vi "Quick Usb Bulk Data Stop Stream.vi"(8 "error in (no error)":errorcluster, 10 "wait":u8, 11 "hDevice":u32) -> (0 "error out":errorcluster, 2 "function return":i32, 3 "hDevice out":u32)   [LabVIEW 2011, in "QuickUSB.lvlib"]
doc: "QUSBLIB QRETURN QuickUsbBulkDataStopStream(\n QHANDLE hDevice,\n QBOOL wait\n);"
uses:
  QuickUSB.lvlib
  QuickUSB.dll
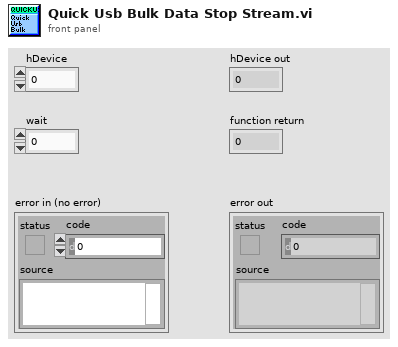
[diagram p1: front panel]
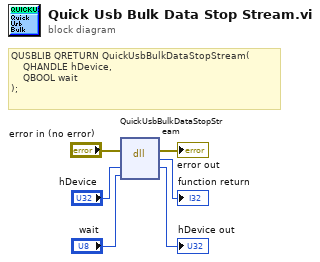
[diagram p0: block diagram]
diagram:
  # "QUSBLIB QRETURN QuickUsbBulkDataStopStream(\n    QHANDLE hDevice,\n    QBOOL wait\n);"
  n1 = dll-call lib="C:/QuickUSB/QuickUSB.*" fn="QuickUsbBulkDataStopStream"(error in="error in (no error)", "hDevice"="hDevice", "wait"="wait") -> (error out=→"error out":errorcluster, →"function return":i32, "hDevice"=→"hDevice out":u32)  [unwired: 3 in, 1 out]
